vi "Read Compiled Settings.vi"(8 "error in (no error)":errorcluster, 11 "Device Reference In":T2 format="%.0x") -> (0 "error out":errorcluster, 1 "Write Block Descriptors":T1[](array[typedef]), 2 "Read Block Descriptors":T1[](array[typedef]), 3 "Device Reference Out":T2 format="%.0x", 4 "Write":bool, 5 "max channel count bytes":u32, 6 "Read":bool)   [LabVIEW 2019, in "RefMem DMA Engine.lvlib"]
uses:
  RefMem DMA Engine.lvlib
  <vilib>/NI VeriStand/Custom Device API/Custom Device Item Ref.ctl
  Shared/Block descriptor.ctl
  Shared/Compiled Settings Typedef.ctl
  Shared/Constants.vi
  <vilib>/NI VeriStand/Custom Device API/Get Item Property (Variant).vi
  <vilib>/NI VeriStand/Custom Device API/Custom Device API.lvlib
  Shared/RefMem DMA Shared.lvlib
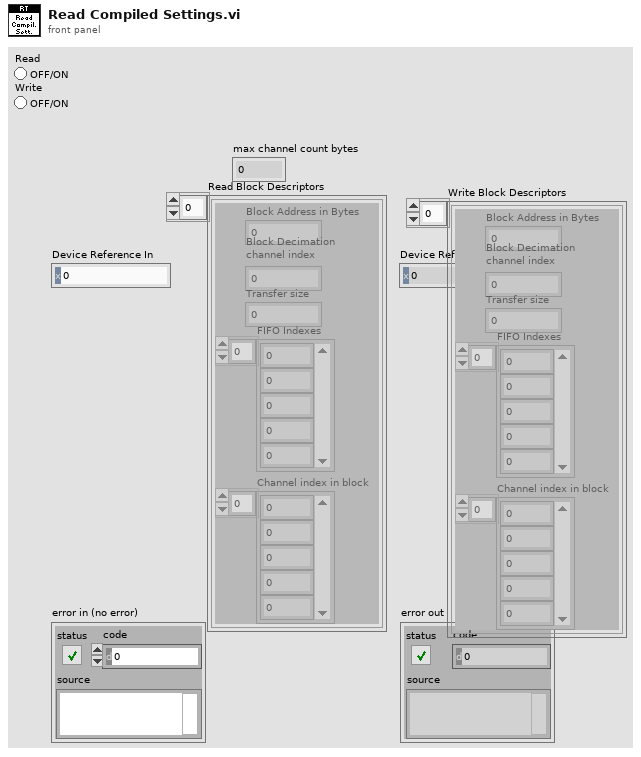
[diagram p1: front panel]
types:
  T1 = typedef "RefMem DMA Shared.lvlib/Block descriptor.ctl" = cluster{"Block Address in Bytes":u32, "Block Decimation \nchannel index":i32, "Transfer size":u32, "FIFO Indexes":i32[], "Channel index in block":i32[]}
  T2 = typedef "Custom Device API.lvlib/Custom Device Item Ref.ctl" = u64
  T3 = typedef "RefMem DMA Shared.lvlib/Compiled Settings Typedef.ctl" = cluster{"Read Block Descriptors":T1[], "max channel count bytes":u32, "Read":bool, "Write":bool, "Write Block Descriptors":T1[]}
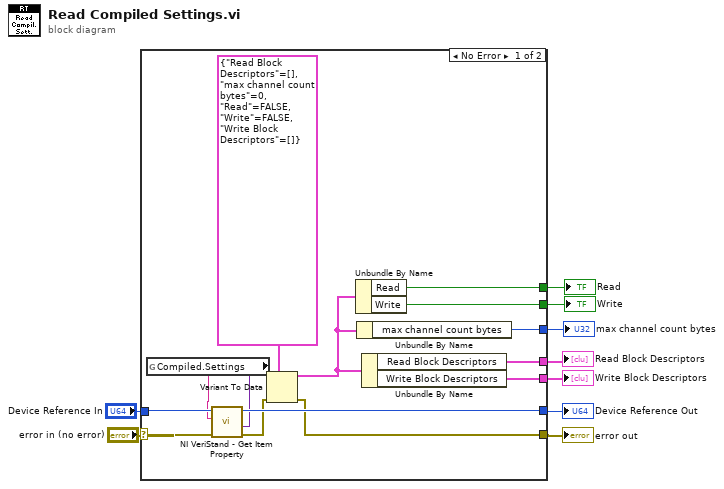
[diagram p0: block diagram]
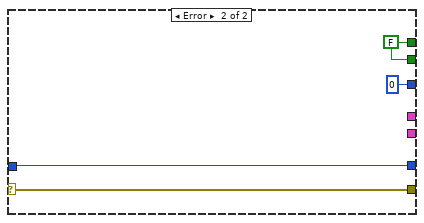
[diagram p2: hidden frame]
diagram:
  n1 = case shown="No Error" "error in (no error)" {
    selector: "error in (no error)" -> [w23 w27]
    tunnel: [w18 w27] -> w8
    tunnel: "Device Reference In" -> [w22 w24]
    tunnel: [w21 w24] -> w6
    tunnel: [w16 w26] -> w5
    tunnel: [w15 w26] -> w4
    tunnel: [w14 u32 0 ("max channel count bytes")] -> w3
    tunnel: [w12 _] -> w2
    tunnel: [w11 _] -> w1
    frame No Error {
      n2 = global read "Constants.vi" "Compiled.Settings"() -> (w10:string)
      n3 = call-poly <vilib>:"NI VeriStand - Get Item Property.vi"("error in (no error)"=w23, "Property Name"=w10, "Item Ref in"=w22) -> ("error out"=w20:errorcluster, "Value"=w19:variant, "Item Ref out"=w21:T2)  [unwired: 5 in, 1 out]
      n4 = Variant To Data(error in=w20, type=T3 {"Read Block Descriptors"=[], "max channel count bytes"=0, "Read"=FALSE, "Write"=FALSE, "Write Block Descriptors"=[]} ("Compiled Settings"), Variant=w19) -> (data=w13:T3, error out=w18:errorcluster)
      n5 = Unbundle By Name(w13) -> ("Read"=w16:bool, "Write"=w15:bool)
      n6 = Unbundle By Name(w13) -> ("max channel count bytes"=w14:u32)
      n7 = Unbundle By Name(w13) -> ("Read Block Descriptors"=w12:T1[], "Write Block Descriptors"=w11:T1[])
    }
    frame Error {
      w26 = FALSE ("Read")
    }
  }
  "error out" <- w8
  "Device Reference Out" <- w6
  "max channel count bytes" <- w3
  "Read" <- w5
  "Write" <- w4
  "Read Block Descriptors" <- w2
  "Write Block Descriptors" <- w1
